vi "ByRef In-Place Blocking.vi"   [LabVIEW 2018]
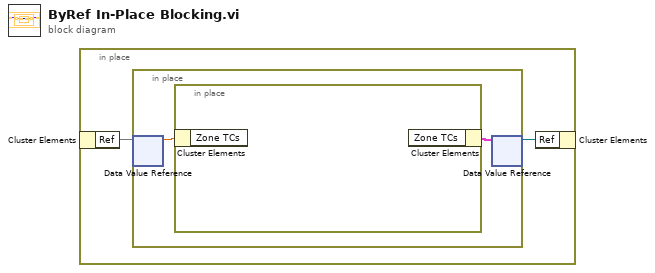
[diagram p0: block diagram]
diagram:
  n1 = in-place {
    n2 = in-place-cluster #1() -> ("Ref"=w2)  [unwired: 1 in]
    n3 = in-place {
      n4 = in-place-dvr #2(w2) -> (w4:dbl)  [unwired: 1 out]
      n5 = in-place {
        n6 = in-place-cluster #3(w4) -> ()  [unwired: 1 out]
        n7 = in-place-cluster #3() -> (w3:cluster{})  [unwired: 1 in]
      }
      n8 = in-place-dvr #2(w3) -> (w1:refnum<data-value>)  [unwired: 1 out]
    }
    n9 = in-place-cluster #1("Ref"=w1) -> ()  [unwired: 1 out]
  }
